vi "R4GetSignals.vi"(7 "LabVIEW Web Service Request":refnum<class "Web Request.lvclass">) -> (3 "R1 Signal Status":T1)   [LabVIEW 2016]
uses:
  <vilib>/wsapi/Web Request.lvclass
  R4Controls/R4Signal_Status.ctl
panel:
  # "Use the Web Service Request input terminal to call the VIs on the Web Services palette. Do not remove it from the connector pane unless you don't need access to the palette."
  # "Each additional control wired to the connector pane will be available as an input in the URL. To include an indicator in terminal-mode output (the default setting), it must also be wired to the connector pane."
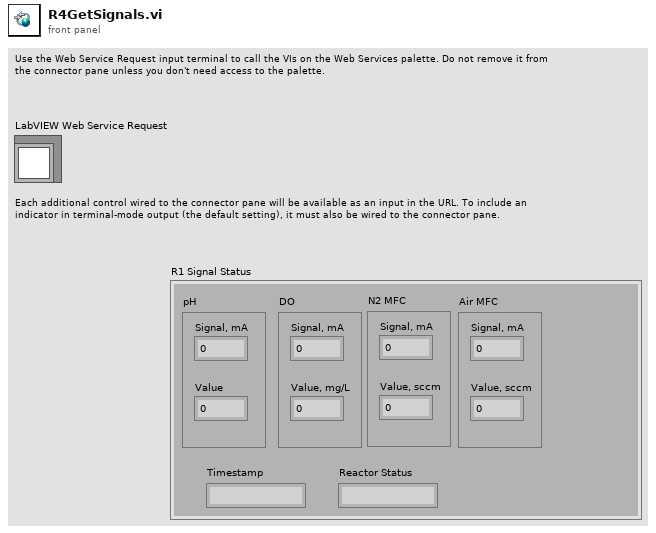
[diagram p1: front panel]
types:
  T1 = typedef "R4Signal_Status.ctl" = cluster{"pH":cluster{"Signal, mA":dbl, "Value":dbl}, "DO":cluster{"Signal, mA":dbl, "Value, mg/L":dbl}, "Timestamp":string, "Reactor Status":string, "N2 MFC":cluster{"Signal, mA":dbl, "Value, sccm":dbl}, "Air MFC":cluster{"Signal, mA":dbl, "Value, sccm":dbl}}
  T2 = cluster{"Signal, mA":dbl, "Value, UNITS HERE":dbl}
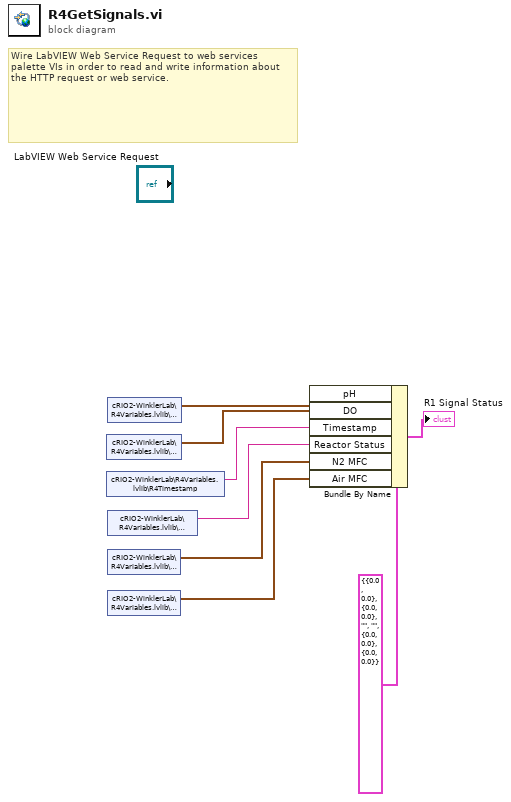
[diagram p0: block diagram]
diagram:
  # "Wire LabVIEW Web Service Request to web services palette VIs in order to read and write information about the HTTP request or web service."
  n1 = shared-variable "cRIO2-WinklerLab\\R4Variables.lvlib\\R4Signals.lvlib\\R4DO"() -> (w5:cluster{"Signal":dbl, "Value":dbl})  [unwired: 1 in, 1 out]
  n2 = shared-variable "cRIO2-WinklerLab\\R4Variables.lvlib\\R4Timestamp"() -> (w4:string)  [unwired: 1 in, 1 out]
  n3 = shared-variable "cRIO2-WinklerLab\\R4Variables.lvlib\\R4Signals.lvlib\\R4pH"() -> (w6:cluster{"Signal":dbl, "Value":dbl})  [unwired: 1 in, 1 out]
  n4 = shared-variable "cRIO2-WinklerLab\\R4Variables.lvlib\\R4Status"() -> (w3:string)  [unwired: 1 in, 1 out]
  n5 = shared-variable "cRIO2-WinklerLab\\R4Variables.lvlib\\R4Signals.lvlib\\R4N2"() -> (w2:cluster{"Signal":dbl, "Value":dbl})  [unwired: 1 in, 1 out]
  n6 = shared-variable "cRIO2-WinklerLab\\R4Variables.lvlib\\R4Signals.lvlib\\R4Air"() -> (w1:T2)  [unwired: 1 in, 1 out]
  n7 = Bundle By Name(cluster=T1 {"pH"={"Signal, mA"=0.0, "Value"=0.0}, "DO"={"Signal, mA"=0.0, "Value, mg/L"=0.0}, "Timestamp"="", "Reactor Status"="", "N2 MFC"={"Signal, mA"=0.0, "Value, sccm"=0.0}, "Air MFC"={"Signal, mA"=0.0, "Value, sccm"=0.0}} ("Signal Status"), "pH"=w6, "DO"=w5, "Timestamp"=w4, "Reactor Status"=w3, "N2 MFC"=w2, "Air MFC"=w1) -> (→"R1 Signal Status":T1)
